vi "_isBufferFull.vi"(11 "VariantBuffer in":refnum<class "VariantBuffer.lvclass">) -> (2 "isFull":bool)   [LabVIEW 2013, in "CircularBuffer.lvlib" / "VariantBuffer.lvclass"]
uses:
  VariantBuffer.lvclass
  VariantBuffer.lvclass/VariantBuffer.ctl
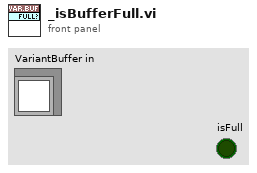
[diagram p1: front panel]
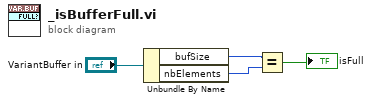
[diagram p0: block diagram]
diagram:
  n1 = Unbundle By Name("VariantBuffer in") -> ("bufSize"=w2:i32, "nbElements"=w3:i32)
  n2 = Equal?(x=w2, y=w3) -> (x = y?=→"isFull":bool)
